vi "Current Mode.vi"   [LabVIEW 2025]
uses:
  <vilib>/Rock Robotics/WPI/Joystick/XBox Axes Indexer.ctl
  <vilib>/Rock Robotics/WPI/Joystick/XBox Buttons Indexer.ctl
  Current Modes.ctl
  <vilib>/Rock Robotics/WPI/Utilities/WPI_GetSetVariantRefNum.vi
  Framework/Robot Global Data.vi
types:
  T1 = typedef "Current Modes.ctl" = u16
  T2 = typedef "XBox Buttons Indexer.ctl" = enum16{"A", "B", "X", "Y", "Left Bumper", "Right Bumper", "Back", "Start", "Left Joystick", "Right Joystick"}
  T3 = typedef "XBox Axes Indexer.ctl" = enum16{"Left X", "Left Y", "Left Trigger", "Right Trigger", "Right X", "Right Y"}
  T4 = typedef "WPI_JoystickDevRef.ctl" = cluster{"Device":T5}
  T5 = typedef "WPI_JoystickDeviceEnum.ctl" = enum16{"USB 0", "USB 1", "USB 2", "USB 3", "USB 4", "USB 5"}
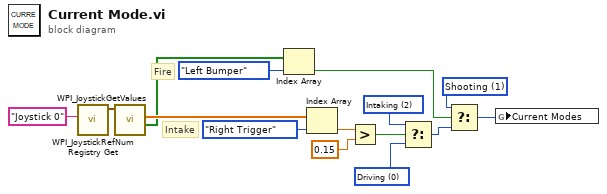
[diagram p0: block diagram]
diagram:
  w3 = T1 1 items=["Driving", "Shooting", "Intaking"] ("t")
  w4 = T1 2 items=["Driving", "Shooting", "Intaking"] ("t")
  w5 = T1 0 items=["Driving", "Shooting", "Intaking"] ("Current Modes")
  # "Fire"
  # "Intake"
  n1 = call <vilib>:"WPI_JoystickRefNum Registry Get.vi"("refnum name"="Joystick 0") -> ("JoystickDevRef"=w2:T4)  [unwired: 1 in, 9 out]
  n2 = call <vilib>:"WPI_JoystickGetValues.vi"("JoystickDevRef"=w2) -> ("Buttons"=w12:bool[], "Axes"=w14:dbl[])  [unwired: 6 in, 3 out]
  n3 = Index Array(array=w12, index=XBox_Buttons_Indexer."Left Bumper" ("XBox Buttons")) -> (element=w6:bool)
  n4 = Index Array(array=w14, index=XBox_Axes_Indexer."Right Trigger" ("XBox Axes")) -> (element=w10:dbl)
  n5 = Greater?(x=w10, y=0.15) -> (0:w8:bool)
  n6 = Select(t=w4, s=w8, f=w5) -> (s? t:f=w7:T1)
  n7 = Select(t=w3, s=w6, f=w7) -> (s? t:f=w1:T1)
  n8 = global write "Robot Global Data.vi" "Current Modes"(w1) -> ()
